vi "Network_Streams_Writer.vi"() -> ()   [LabVIEW 2014]
uses:
  <resource>/objmgr/ni.dex.rc
panel:
  out "Error":bool
  out "Is Connected":bool
  in  "stop":bool
  in  "data in":string
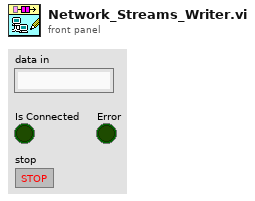
[diagram p1: front panel]
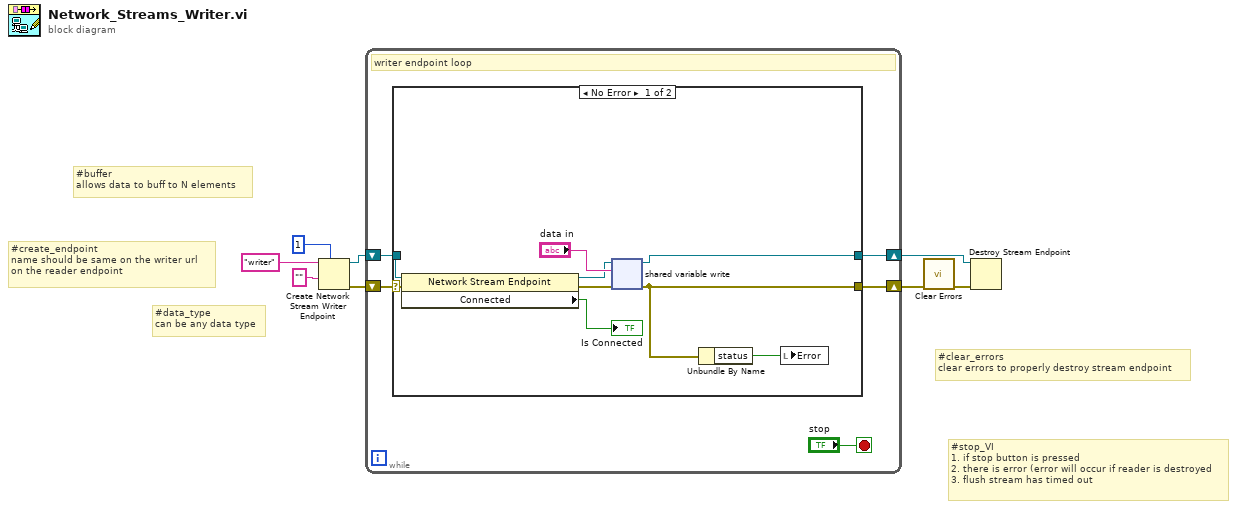
[diagram p0: block diagram]
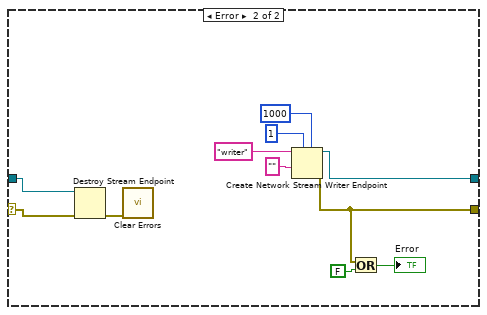
[diagram p2: hidden frame]
diagram:
  # "#clear_errors\nclear errors to properly destroy stream endpoint"
  # "#stop_VI\n1. if stop button is pressed\n2. there is error (error will occur if reader is destroyed\n3. flush stream has timed out"
  # "#buffer\nallows data to buff to N elements"
  # "#data_type\ncan be any data type"
  # "#create_endpoint\nname should be same on the writer url\non the reader endpoint"
  n1 = Create Network Stream Writer Endpoint(7:1 ("writer buffer size"), 9:"" ("writer name"), 11:"writer" ("writer name")) -> (0:w8:errorcluster, 3:w7:refnum<k21>)  [unwired: 4 in]
  n2 = while {
    shift-right: [w13] -> w4
    shift-left: w7 -> [w12]
    shift-right: [w10] -> w2
    shift-left: w8 -> [w11]
    stop <- "stop" stop-if-true
    # "writer endpoint loop"
    n3 = case shown="No Error" w11 {
      selector: w11 -> [w17 w32]
      tunnel: [w22 w26] -> w13
      tunnel: w12 -> [w19 w33]
      tunnel: [w15 w24] -> w10
      frame No Error {
        n4 = property class="Network Stream Endpoint"(reference=w19, error in=w17) -> (reference out=w20:refnum<k21>, error out=w18:errorcluster, "Connected"=→"Is Connected":bool)
        n5 = shared-variable-write(w20, w18, "data in") -> (w22:refnum<k21>, w15:errorcluster)  [unwired: 1 in, 1 out]
        n6 = Unbundle By Name(w15) -> ("status"=w14:bool)
        n7 = local write "Error"(w14) -> ()
      }
      frame Error {
        n8 = Destroy Stream Endpoint(8:w32, 11:w33) -> (0:w31:errorcluster)
        n9 = call <vilib>:"Clear Errors.vi"("error in (no error)"=w31) -> ()  [unwired: 5 in, 2 out]
        n10 = Create Network Stream Writer Endpoint(5:1000 ("timeout in ms (-1)"), 7:1 ("writer buffer size"), 9:"" ("writer name"), 11:"writer" ("writer name")) -> (0:w24:errorcluster, 3:w26:refnum<k21>)  [unwired: 3 in]
        n11 = Or(x=w24, y=FALSE) -> (x .or. y?=→"Error":bool)
      }
    }
  }
  n12 = call <vilib>:"Clear Errors.vi"("error in (no error)"=w2) -> ("error out"=w1:errorcluster)  [unwired: 5 in, 1 out]
  n13 = Destroy Stream Endpoint(8:w1, 11:w4) -> ()  [unwired: 1 out]
